vi "Encode LEN.vi"(10 "Data":u8[](array[numeric]) format="%.0x", 11 "Buffer in":u8[](array[numeric]) format="%.0x") -> (3 "Buffer":u8[](array[numeric]) format="%.0x")   [LabVIEW 2020, in "LV-Proto.lvlib"]
uses:
  LV-Proto.lvlib
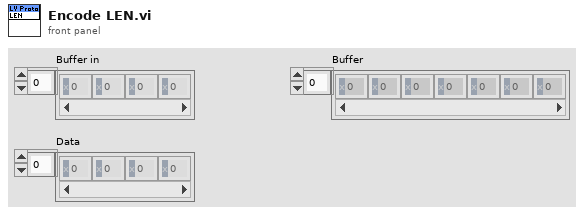
[diagram p1: front panel]
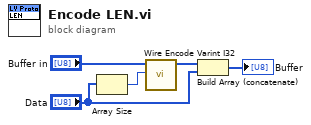
[diagram p0: block diagram]
diagram:
  n1 = Array Size(array="Data") -> (size(s)=w5:i32)
  n2 = call "Wire Encode Varint I32.vi"("I32"=w5, "Buffer in"="Buffer in") -> ("Buffer"=w3:u8[])  [unwired: 9 in]
  n3 = Build Array (concatenate)(w3, "Data") -> (→"Buffer":u8[])
